vi "Perspective Distortion Loop.vi"(7 "Open File Path":path, 8 "Error In":errorcluster, 10 "Live Button":bool, 11 "Stop (F)":bool) -> (0 "Error Out":errorcluster, 1 "Image Index":dbl, 3 "Left Image in":T1(plugin-control), 4 "Gauge":cluster{dbl, dbl}(knob) scale=0.0..50.0, 5 "Time Stamp":timestamp)   [LabVIEW 2012]
uses:
  <vilib>/Platform/TimedLoop/XDataNode/timing_clust.ctl
  <vilib>/Platform/TimedLoop/XDataNode/nitl_modes.ctl
  <vilib>/Platform/TimedLoop/XDataNode/wakeup.ctl
  <vilib>/platform/TimedLoop/XDataNode/XDataNode.xnode
  <vilib>/Platform/TimedLoop/XDataNode/XDNodeRunTimeDep.lvlib
panel:
  in  "Perspective Button":bool
  out "Iteration Duration":i64
  in  "Calibration File Left":path=path "C:/Users/whitemrj/Desktop/New folder/pizza cal Left.png"
  in  "Calibration File Right":path=path "C:/Users/whitemrj/Desktop/New folder/pizza cal Right.png"
  in  "Record Button":bool
  in  "Save File Path":path=path "C:/Users/whitemrj/Desktop/New folder"
  out "Right Image out":T1(plugin-control)
  out "Left Image out":T1(plugin-control)
  out "Right Image in":T1(plugin-control)
  out "Image Type":T2 items=["Grayscale (U8)", "Grayscale (I16)", "Grayscale (SGL)", "Complex (CSG)", "RGB (U32)", "HSL (U32)", "RGB (U64)", "Grayscale (U16)"]
  out "Y Resolution":i32
  out "X Resolution":i32
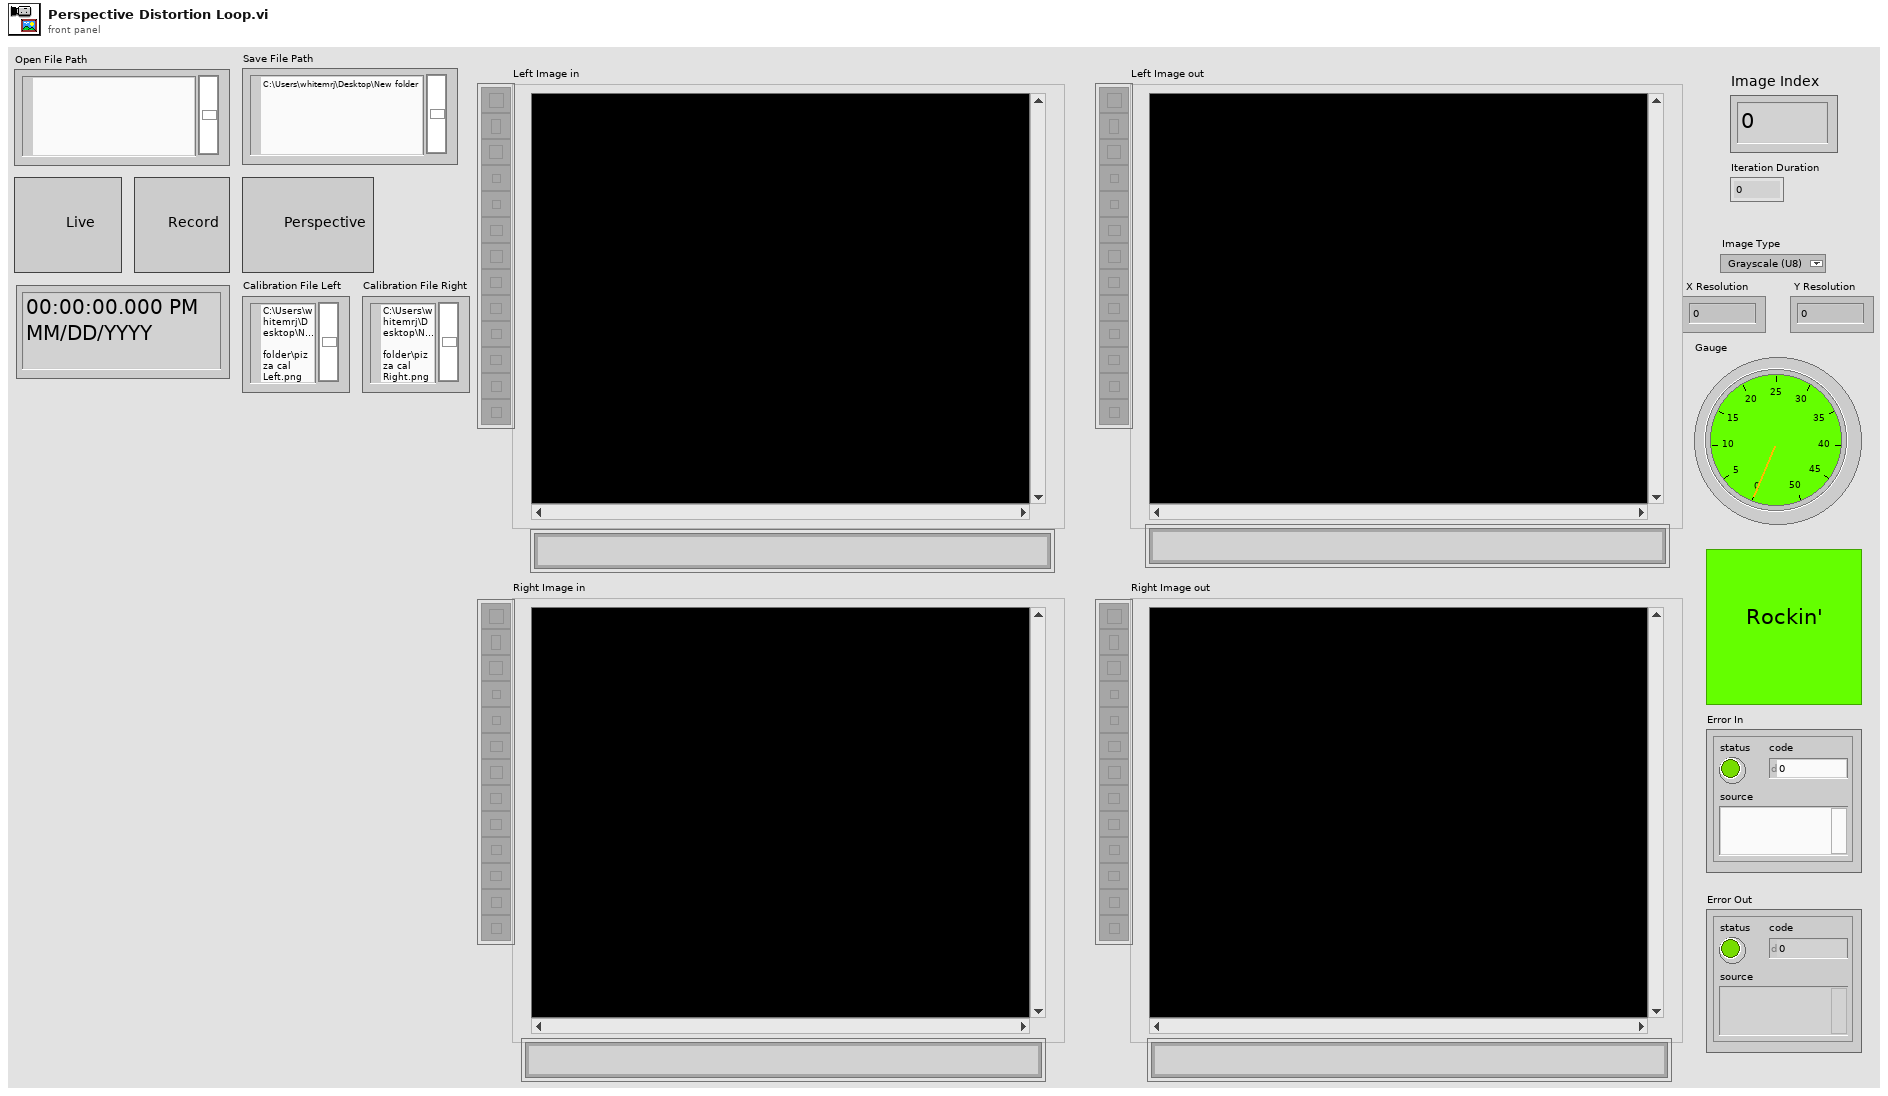
[diagram p1: front panel]
types:
  T1 = typedef "IMAQ Image.ctl" = refnum<image>
  T2 = typedef "Image Type" = u32
  T3 = typedef "XDNodeRunTimeDep.lvlib/timing_clust.ctl" = cluster{"Expected End [f-1]":u64, "Actual End [f-1]":u64, "Finished Late? [f-1]":bool, "Expected End [i-1]":u64, "Actual End [i-1]":u64, "Finished Late? [i-1]":bool, "Expected Start [i]":u64, "Actual Start [i]":u64, "Expected Start [f]":u64, "Actual Start [f]":u64, "Source Name":string, "Structure Name":string, "Period":i64, "Deadline":i64, "Offset":i64, "Start":i64, "Priority":i32, "Timeout":i32, "Mode":T4, "Wakeup Reason":T5, "Error":errorcluster, "Source Type":string, "Secondary Source Type":string, "Global End Time":u64, "Global Start Time":u64, "Frame Duration":u64, "Iteration Duration":u64, "Assigned CPU":i32, "I/O Scan Engine Mode":u32}
  T4 = typedef "XDNodeRunTimeDep.lvlib/nitl_modes.ctl" = enum32{"No Change", "Process missed periods, maintain original phase", "Discard missed periods, maintain original phase", "Process missed periods, ignore original phase", "Discard missed periods, ignore original phase"}
  T5 = typedef "XDNodeRunTimeDep.lvlib/wakeup.ctl" = enum32{"Normal", "Aborted", "Asynchronous wakeup", "Timing source error", "Timed loop error", "Timeout"}
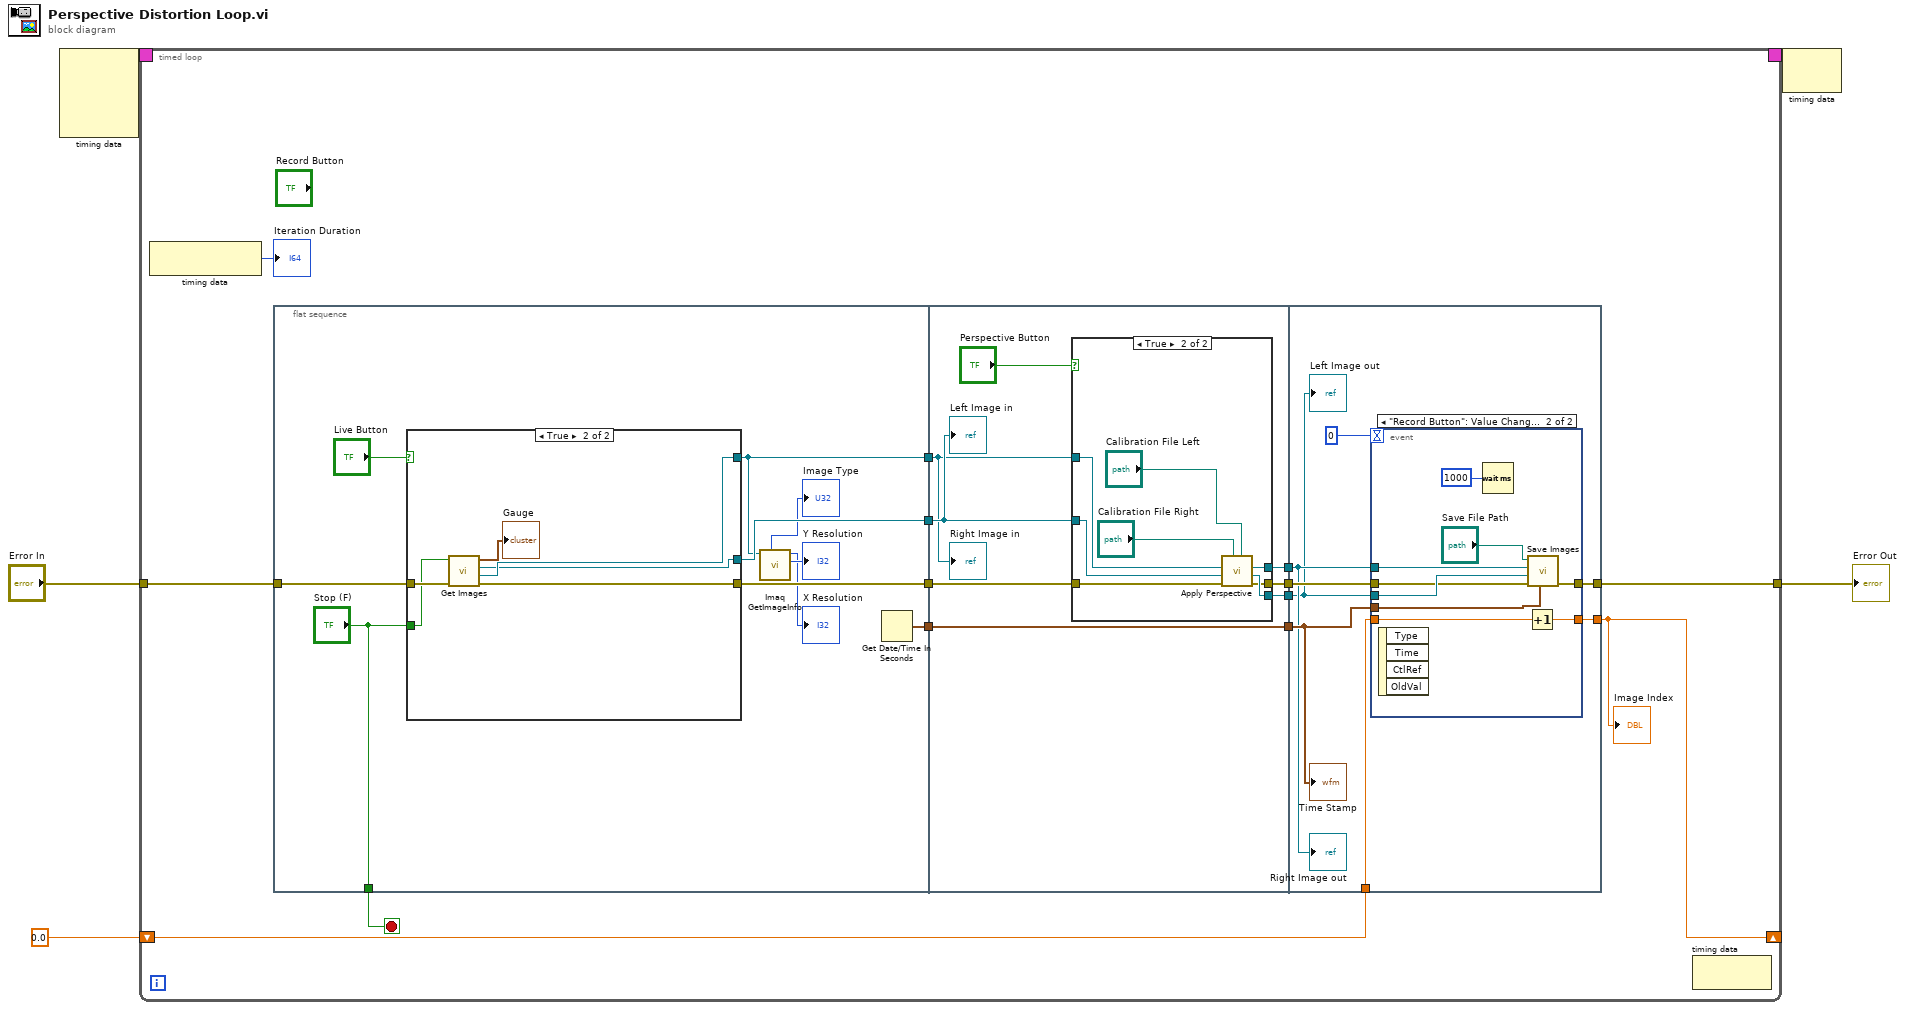
[diagram p0: block diagram]
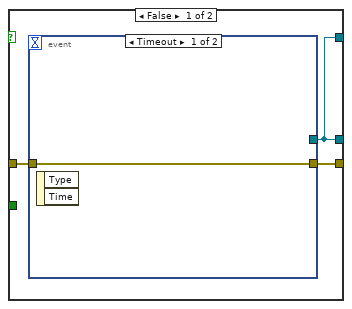
[diagram p2: hidden frame]
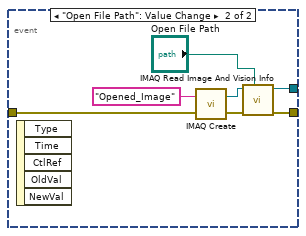
[diagram p3: hidden frame]
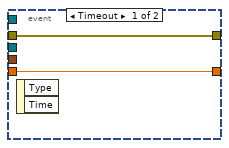
[diagram p5: hidden frame]
diagram:
  n1 = node-c288() -> (w5:T3)  [unwired: 4 in]
  n2 = timed-loop {
    timing: w5 -> [_]
    timing-out: [_] -> w4
    tunnel: "Error In" -> [w17]
    tunnel: [w6] -> w2
    shift-right: [w12] -> _
    shift-left: 0.0 ("Image Index") -> [w13]
    stop <- w18 stop-if-true
    n3 = node-c288() -> (→"Iteration Duration":i64)  [unwired: 1 in]
    n4 = flat-sequence {
      tunnel: ["Stop (F)"] -> w18
      tunnel: w17 -> [w27]
      tunnel: [w20] -> w16
      tunnel: [w26] -> w15
      tunnel: [w25] -> w14
      tunnel: [w24] -> w7
      tunnel: w16 -> [w50]
      tunnel: w15 -> [w52]
      tunnel: w14 -> [w53]
      tunnel: [w51] -> w11
      tunnel: [w49] -> w10
      tunnel: [w48] -> w9
      tunnel: [w47] -> w8
      tunnel: w7 -> [w47]
      tunnel: w13 -> [w73]
      tunnel: [w72] -> w12
      tunnel: w11 -> [w71]
      tunnel: w10 -> [w68]
      tunnel: w9 -> [w67]
      tunnel: w8 -> [w70]
      tunnel: [w69] -> w6
      frame #0 {
        n5 = case shown="True" "Live Button" {
          tunnel: w27 -> [w30 w46]
          tunnel: [w31 w45] -> w25
          tunnel: [w32 w44] -> w20
          tunnel: "Stop (F)" -> [_ w43]
          tunnel: [w32 w42] -> w26
          frame False {
            n6 = event shown="[0] Timeout" {
              selector: _ -> [_ _]
              dyn-events: _ -> [_ _]
              timeout: _ -> [_ _]
              tunnel: [_ w39] -> w32
              tunnel: [w33 w38] -> w31
              tunnel: w30 -> [w33 w35]
              event Timeout {
                n7 = event-data() -> ()  [unwired: 1 in, 2 out]
              }
              event "Open File Path": Value Change {
                n8 = event-data() -> ()  [unwired: 1 in, 5 out]
                n9 = call "IMAQ Create"("Image Name"="Opened_Image", "error in (no error)"=w35) -> ("New Image"=w37:T1, "error out"=w36:errorcluster)  [unwired: 3 in]
                n10 = call "IMAQ Read Image And Vision Info"("File Path"="Open File Path", "error in (no error)"=w36, "Image"=w37) -> ("error out"=w38:errorcluster, "Image Out"=w39:T1)  [unwired: 6 in, 1 out]
              }
            }
          }
          frame True {
            n11 = call "Get Images.vi"("error in"=w46, "Stop (F)"=w43) -> ("error out"=w45:errorcluster, "Left Image out"=w44:T1, "Right Image out"=w42:T1, "Gauge"=→"Gauge":cluster{dbl, dbl})  [unwired: 6 in]
          }
        }
        n12 = call "Imaq GetImageInfo"("Image"=w20) -> ("Y Resolution"=→"Y Resolution":i32, "X Resolution"=→"X Resolution":i32, "Image Type"=→"Image Type":T2)  [unwired: 3 in, 5 out]
        n13 = Get Date/Time In Seconds() -> (seconds since 1Jan1904=w24:timestamp)
      }
      frame #1 {
        n14 = case shown="True" "Perspective Button" {
          tunnel: w53 -> [w55 w65]
          tunnel: w52 -> [w56 w64]
          tunnel: w50 -> [w57 w63]
          tunnel: [w56 w62] -> w48
          tunnel: [w57 w61] -> w49
          tunnel: [w55 w58] -> w51
          frame False {
          }
          frame True {
            n15 = call "Apply Perspective.vi"("File Path (Image Calibration Left)"="Calibration File Left", "File Path (Image Calibration Right)"="Calibration File Right", "error in"=w65, "Left Image in"=w64, "Right Image in"=w63) -> ("error out"=w58:errorcluster, "Left Image out"=w62:T1, "Right Image out"=w61:T1)  [unwired: 4 in]
          }
        }
        "Left Image in" <- w52
        "Right Image in" <- w50
      }
      frame #2 {
        n16 = event shown="[1] \"Record Button\": Value Change" {
          selector: _ -> [_ _]
          dyn-events: _ -> [_ _]
          timeout: 0 -> [_ _]
          tunnel: w70 -> [_ w81]
          tunnel: [w74 w84] -> w69
          tunnel: [w75 w82] -> w72
          tunnel: w73 -> [w75 w83]
          tunnel: w67 -> [_ w79]
          tunnel: w68 -> [_ w78]
          tunnel: w71 -> [w74 w76]
          event Timeout {
            n17 = event-data() -> ()  [unwired: 1 in, 2 out]
          }
          event "Record Button": Value Change {
            n18 = event-data() -> ()  [unwired: 1 in, 4 out]
            n19 = Wait (ms)(milliseconds to wait=u32 1000) -> ()  [unwired: 1 out]
            n20 = Increment(x=w83) -> (x+1=w82:dbl)
            n21 = call "Save Images.vi"("Time Stamp"=w81, "error in (no error)"=w76, "Left Image"=w79, "Right Image"=w78, "Save File Path"="Save File Path") -> ("error out"=w84:errorcluster)  [unwired: 6 in]
          }
        }
        "Left Image out" <- w67
        "Right Image out" <- w68
        "Time Stamp" <- w70
      }
    }
    n22 = node-c288() -> ()  [unwired: 1 in, 1 out]
    "Image Index" <- w12
  }
  "Error Out" <- w2
  n23 = node-c288(w4) -> ()  [unwired: 1 out]
